vi "CrabWalk.vi"(7 "Speed (m/s)":dbl=0.2, 8 "error in\n(no error)":errorcluster, 9 "Front Rotate (degree)":dbl, 10 "Distance Y (m)":dbl=0.3, 11 "Distance X (m)":dbl=0.3) -> (0 "error out":errorcluster, 3 "Duration (ms)":dbl)   [LabVIEW 2017]
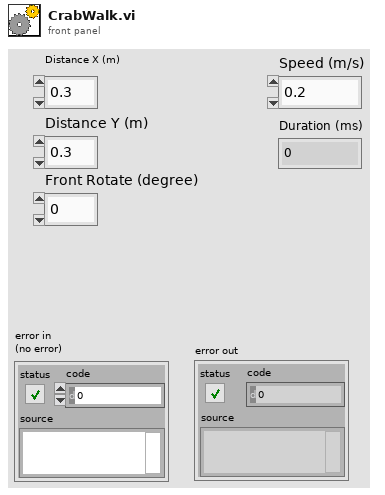
[diagram p1: front panel]
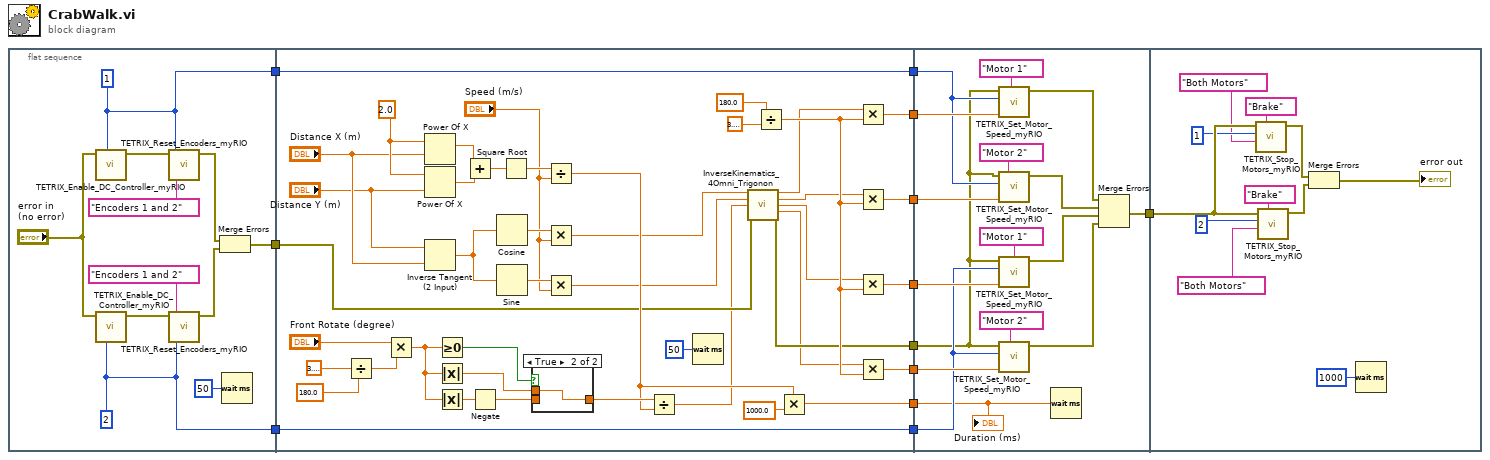
[diagram p0: block diagram]
diagram:
  n1 = flat-sequence {
    tunnel: [w17] -> w12
    tunnel: [w14] -> w11
    tunnel: [w13] -> w10
    tunnel: w12 -> [w33]
    tunnel: w11 -> [w51]
    tunnel: w10 -> [w50]
    tunnel: [w45] -> w8
    tunnel: [w51] -> w7
    tunnel: [w32] -> w6
    tunnel: [w50] -> w5
    tunnel: [w49] -> w4
    tunnel: [w44] -> w3
    tunnel: [w43] -> w2
    tunnel: [w42] -> w1
    tunnel: [w70] -> w9
    tunnel: w8 -> [w81]
    tunnel: w7 -> [w77]
    tunnel: w6 -> [w71]
    tunnel: w5 -> [w72]
    tunnel: w4 -> [w69]
    tunnel: w3 -> [w79]
    tunnel: w2 -> [w74]
    tunnel: w1 -> [w76]
    tunnel: w9 -> [w94]
    frame #0 {
      w13 = u8 1 ("Controller ID#  (I2C Address)")
      w14 = u8 2 ("Controller ID#  (I2C Address)")
      n2 = call <vilib>:"TETRIX_Enable_DC_Controller_myRIO.vi"("Controller ID#  (I2C Address)"=w13, "Error/Flow In"="error in\n(no error)") -> ("Error/Flow Out"=w22:errorcluster)  [unwired: 5 in]
      n3 = call <vilib>:"TETRIX_Enable_DC_Controller_myRIO.vi"("Controller ID#  (I2C Address)"=w14, "Error/Flow In"="error in\n(no error)") -> ("Error/Flow Out"=w23:errorcluster)  [unwired: 5 in]
      n4 = call <vilib>:"TETRIX_Reset_Encoders_myRIO.vi"("Select Encoder"="Encoders 1 and 2", "Controller ID#  (I2C Address)"=w13, "Error/Flow In"=w22) -> ("Error/Flow Out"=w19:errorcluster)  [unwired: 4 in]
      n5 = call <vilib>:"TETRIX_Reset_Encoders_myRIO.vi"("Select Encoder"="Encoders 1 and 2", "Controller ID#  (I2C Address)"=w14, "Error/Flow In"=w23) -> ("Error/Flow Out"=w18:errorcluster)  [unwired: 4 in]
      n6 = Merge Errors(w19, w18) -> (w17:errorcluster)
      n7 = Wait (ms)(milliseconds to wait=u32 50) -> ()  [unwired: 1 out]
    }
    frame #1 {
      w65 = 2.0 ("y")
      n8 = Divide(x=3.141592653589793, y=180.0) -> (x/y=w57:dbl)
      n9 = Multiply(x="Front Rotate (degree)", y=w57) -> (x*y=w35:dbl)
      n10 = Power Of X(1:"Distance X (m)", 2:w65) -> (0:w64:dbl)
      n11 = Power Of X(1:"Distance Y (m)", 2:w65) -> (0:w63:dbl)
      n12 = Inverse Tangent (2 Input)(1:"Distance X (m)", 2:"Distance Y (m)") -> (0:w40:dbl)
      n13 = Greater Or Equal To 0?(x=w35) -> (x >= 0?=w34:bool)
      n14 = Absolute Value(x=w35) -> (abs(x)=w53:dbl)
      n15 = Absolute Value(x=w35) -> (abs(x)=w55:dbl)
      n16 = Add(x=w64, y=w63) -> (x+y=w66:dbl)
      n17 = Negate(x=w55) -> (-x=w54:dbl)
      n18 = Cosine(x=w40) -> (cos(x)=w61:dbl)
      n19 = Sine(x=w40) -> (sin(x)=w60:dbl)
      n20 = Square Root(x=w66) -> (sqrt(x)=w62:dbl)
      n21 = case shown="True" w34 {
        tunnel: w53 -> [_ w68]
        tunnel: w54 -> [w67 _]
        tunnel: [w67 w68] -> w52
        frame False {
        }
        frame True {
        }
      }
      n22 = Divide(x=w62, y="Speed (m/s)") -> (x/y=w36:dbl)
      n23 = Multiply(x=w61, y="Speed (m/s)") -> (x*y=w25:dbl)
      n24 = Multiply(x=w60, y="Speed (m/s)") -> (x*y=w26:dbl)
      n25 = Divide(x=w52, y=w36) -> (x/y=w27:dbl)
      n26 = Wait (ms)(milliseconds to wait=u32 50) -> ()  [unwired: 1 out]
      n27 = call "InverseKinematics_4Omni_Trigonon.vi"("VX"=w25, "VY"=w26, "Omega"=w27, "error in (no error)"=w33) -> ("W1-FL"=w28:dbl, "W2-BL"=w29:dbl, "W3-FR"=w30:dbl, "W4-BR"=w31:dbl, "error out"=w32:errorcluster)  [unwired: 7 in]
      n28 = Divide(x=180.0, y=3.141592653589793) -> (x/y=w41:dbl)
      n29 = Multiply(x=w36, y=1000.0) -> (x*y=w49:dbl)
      n30 = Multiply(x=w28, y=w41) -> (x*y=w43:dbl)
      n31 = Multiply(x=w29, y=w41) -> (x*y=w42:dbl)
      n32 = Multiply(x=w30, y=w41) -> (x*y=w44:dbl)
      n33 = Multiply(x=w31, y=w41) -> (x*y=w45:dbl)
    }
    frame #2 {
      n34 = call <vilib>:"TETRIX_Set_Motor_Speed_myRIO.vi"("Constant Speed (Degrees per second). Sign (+/-)  sets direction."=w74, "Select Channel"="Motor 1", "Controller ID#  (I2C Address)"=w72, "Error/Flow In"=w71) -> ("Error/Flow Out"=w82:errorcluster)  [unwired: 3 in]
      n35 = call <vilib>:"TETRIX_Set_Motor_Speed_myRIO.vi"("Constant Speed (Degrees per second). Sign (+/-)  sets direction."=w76, "Select Channel"="Motor 2", "Controller ID#  (I2C Address)"=w72, "Error/Flow In"=w71) -> ("Error/Flow Out"=w83:errorcluster)  [unwired: 3 in]
      n36 = call <vilib>:"TETRIX_Set_Motor_Speed_myRIO.vi"("Constant Speed (Degrees per second). Sign (+/-)  sets direction."=w79, "Select Channel"="Motor 1", "Controller ID#  (I2C Address)"=w77, "Error/Flow In"=w71) -> ("Error/Flow Out"=w84:errorcluster)  [unwired: 3 in]
      n37 = call <vilib>:"TETRIX_Set_Motor_Speed_myRIO.vi"("Constant Speed (Degrees per second). Sign (+/-)  sets direction."=w81, "Select Channel"="Motor 2", "Controller ID#  (I2C Address)"=w77, "Error/Flow In"=w71) -> ("Error/Flow Out"=w85:errorcluster)  [unwired: 3 in]
      n38 = Wait (ms)(milliseconds to wait=w69) -> ()  [unwired: 1 out]
      n39 = Merge Errors(w82, w83, w84, w85) -> (w70:errorcluster)
      "Duration (ms)" <- w69
    }
    frame #3 {
      n40 = call <vilib>:"TETRIX_Stop_Motors_myRIO.vi"("Stop Mode"="Brake", "Select Channel"="Both Motors", "Controller ID#  (I2C Address)"=u8 1, "Error/Flow In"=w94) -> ("Error/Flow Out"=w96:errorcluster)  [unwired: 3 in]
      n41 = call <vilib>:"TETRIX_Stop_Motors_myRIO.vi"("Stop Mode"="Brake", "Select Channel"="Both Motors", "Controller ID#  (I2C Address)"=u8 2, "Error/Flow In"=w94) -> ("Error/Flow Out"=w95:errorcluster)  [unwired: 3 in]
      n42 = Merge Errors(w96, w95) -> (→"error out":errorcluster)
      n43 = Wait (ms)(milliseconds to wait=u32 1000) -> ()  [unwired: 1 out]
    }
  }
